vi "Read 1D Array I16.vi"(8 "error in (no error)":errorcluster, 9 "start index (0)":i64, 10 "number of elements":i64, 11 "pointer in":u64) -> (0 "error out":errorcluster, 2 "value":i16[](array[numeric]), 3 "pointer out":u64)   [LabVIEW 2013, in "Linux RT IPC.lvlib" / "Shared Memory.lvlib"]
uses:
  Shared Memory.lvlib
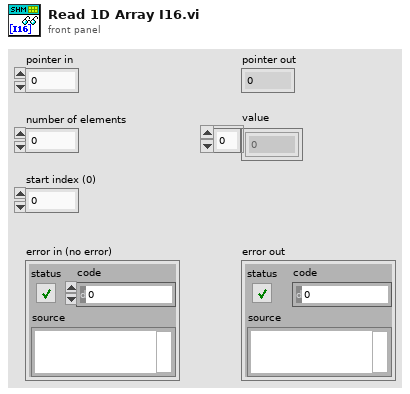
[diagram p1: front panel]
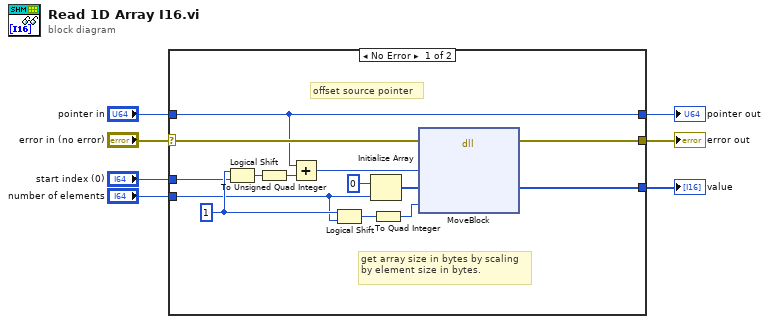
[diagram p0: block diagram]
diagram:
  n1 = case shown="No Error" "error in (no error)" {
    selector: "error in (no error)" -> [w13 w23]
    tunnel: [w12 w23] -> w7
    tunnel: "pointer in" -> [w11 w22]
    tunnel: [w11 w22] -> w4
    tunnel: "number of elements" -> [w9 _]
    tunnel: "start index (0)" -> [w10 _]
    tunnel: [w8 _] -> w1
    frame No Error {
      w14 = i16 1 ("y")
      # "get array size in bytes by scaling by element size in bytes."
      # "offset source pointer"
      n2 = Logical Shift(y=w14, x=w10) -> (x << y=w20:i64)
      n3 = To Unsigned Quad Integer(1:w20) -> (0:w19:u64)
      n4 = Add(x=w11, y=w19) -> (x+y=w15:u64)
      n5 = Logical Shift(y=w14, x=w9) -> (x << y=w21:i64)
      n6 = Initialize Array(i16 0, w9) -> (w17:i16[])
      n7 = To Quad Integer(1:w21) -> (0:w16:i64)
      n8 = dll-call lib="LabVIEW" fn="MoveBlock"(error in=w13, "pointer"=w15, "data"=w17, "size"=w16) -> (error out=w12:errorcluster, "data"=w8:i16[])  [unwired: 5 in, 1 out]
    }
    frame Error {
    }
  }
  "error out" <- w7
  "pointer out" <- w4
  "value" <- w1
